vi "invers kinematic wire.vi"(0 "K":dbl, 7 "phi":dbl, 11 "s":dbl) -> (4 "L1":dbl, 8 "L 2":dbl, 15 "L 3":dbl)   [LabVIEW 2019]
uses:
  <vilib>/imath/engines/lvmath2/RunTimeEngine/Managers/WorkSpace/UID Generator.vi
  <vilib>/imath/engines/lvmath2/RunTimeEngine/RunTimeType/NIMS_RunTimeType_From StrictType (excl LVString).vi
  <instcachedir>/0/NIMS_RunTimeType_From StrictType (excl LVString)_D8AFBA86A94845AAA577C895450664BD.lvgen/NIMS_RunTimeType_From StrictType (excl LVString)_D8AFBA86A94845AAA577C895450664BD_000.vi
  <vilib>/imath/engines/lvmath2/RunTimeEngine/LocalVariableDefStatement/MC_LocalVariableDefStatement_Display.vi
  <vilib>/imath/engines/lvmath2/RunTimeEngine/Managers/SymbolTable/Clear UID.vi
  <vilib>/imath/engines/lvmath2/RunTimeEngine/NodeEndStatement/NIMS_NodeEndStatement_Output.vi
  <instcachedir>/0/NIMS_NodeEndStatement_Output_53EC0D466D134D7ABD903AC30B43404B.lvgen/NIMS_NodeEndStatement_Output_53EC0D466D134D7ABD903AC30B43404B_001.vi
  <vilib>/imath/engines/lvmath2/RunTimeEngine/ErrorHandling/NIMS_Finalize Error.vi
  <vilib>/imath/engines/lvmath2/RunTimeEngine/Managers/SymbolTable/NIMS_WorkSpace.lvlib
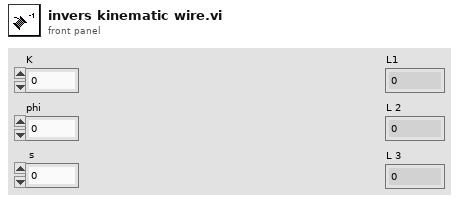
[diagram p1: front panel]
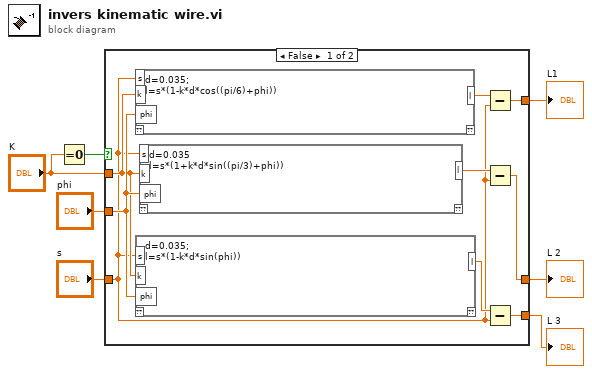
[diagram p0: block diagram]
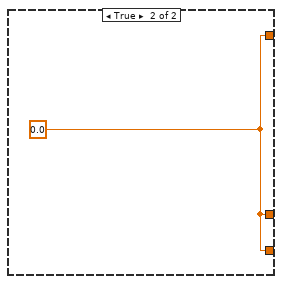
[diagram p2: hidden frame]
diagram:
  n1 = Equal To 0?(x="K") -> (x = 0?=w7:bool)
  n2 = case shown="False" w7 {
    tunnel: [w9 w189] -> w6
    tunnel: "s" -> [w11 _]
    tunnel: [w10 w189] -> w4
    tunnel: [w13 w189] -> w3
    tunnel: "K" -> [w15 _]
    tunnel: "phi" -> [w16 _]
    frame False {
      n3 = mathscript code="d=0.035;\nl=s*(1-k*d*cos((pi/6)+phi))"("s"=w11, "k"=w15, "phi"=w16) -> ("l"=w8:dbl)  [unwired: 1 in, 1 out]
      n4 = mathscript code="d=0.035;\nl=s*(1-k*d*sin(phi))"("s"=w11, "k"=w15, "phi"=w16) -> ("l"=w14:dbl)  [unwired: 1 in, 1 out]
      n5 = mathscript code="d=0.035\nl=s*(1+k*d*sin((pi/3)+phi))"("s"=w11, "k"=w15, "phi"=w16) -> ("l"=w12:dbl)  [unwired: 1 in, 1 out]
      n6 = Subtract(x=w8, y=w11) -> (x-y=w9:dbl)
      n7 = Subtract(x=w12, y=w11) -> (x-y=w10:dbl)
      n8 = Subtract(x=w14, y=w11) -> (x-y=w13:dbl)
    }
    frame True {
      w189 = 0.0
    }
  }
  "L1" <- w6
  "L 2" <- w4
  "L 3" <- w3
